vi "Open Reader Reference.vi"(8 "error in":errorcluster, 11 "TDMS in":refnum<class "TDMS.lvclass">) -> (0 "error out":errorcluster, 3 "TDMS out":refnum<class "TDMS.lvclass">)   [LabVIEW 2019, in "TDMS.lvlib" / "TDMS.lvclass"]
uses:
  TDMS.lvclass
  C:/Users/Public/Documents/Development/builds/Tools/Report.lvlibp/Report.lvclass
  TDMS.lvclass/TDMS.ctl
  Accessors/Write TDMS Read Ref.vi
  builds/Tools/Report.lvlibp/Accessors/Read Report Path.vi
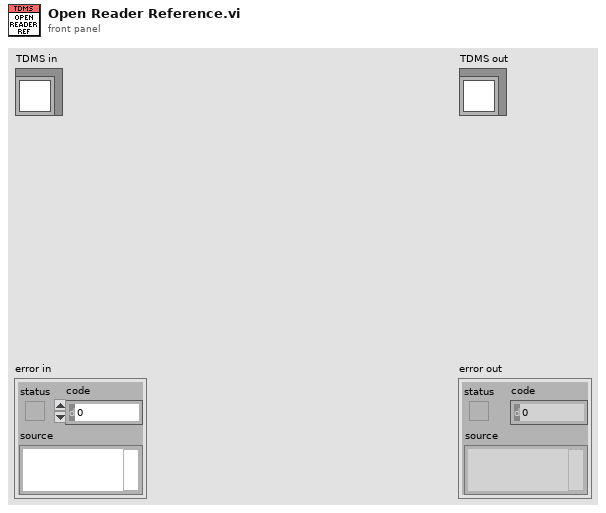
[diagram p1: front panel]
types:
  T1 = enum16{"open", "open or create", "create or replace", "create", "open (read-only)"}
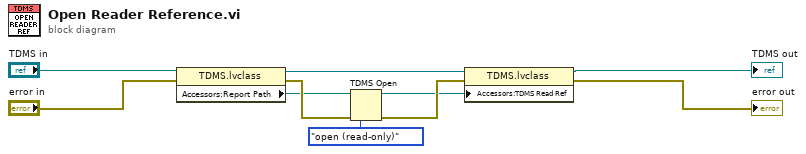
[diagram p0: block diagram]
diagram:
  n1 = property class="TDMS.lvclass"(reference="TDMS in", error in="error in") -> (reference out=w8:refnum<class "TDMS.lvclass">, error out=w7:errorcluster, "Accessors:Report Path"=w5:path)
  n2 = TDMS Open(8:w7, 10:T1."open (read-only)" ("operation (0:open)"), 11:w5) -> (0:w10:errorcluster, 3:w9:refnum<k34>)  [unwired: 4 in]
  n3 = property class="TDMS.lvclass"(reference=w8, error in=w10, "Accessors:TDMS Read Ref"=w9) -> (reference out=→"TDMS out":refnum<class "TDMS.lvclass">, error out=→"error out":errorcluster)
